vi "stimulus.vi"(7 "幅值(V)":dbl, 8 "stop frequency [Hz]":dbl, 9 "start frequency [Hz]":dbl, 10 "信号时长":dbl, 11 "Format":cluster{"Rate":i32, "Bits":i32, "Channels":u32}={"Rate"=44100, "Bits"=32, "Channels"=2}) -> (2 "Buffer size":i32, 3 "Output data":i32[][](array[numeric]))   [LabVIEW 2018]
uses:
  <vilib>/addons/_NISVFA/_Generation/SoundVib_Generation.lvlib
panel:
  in  "信号时长(s)":dbl
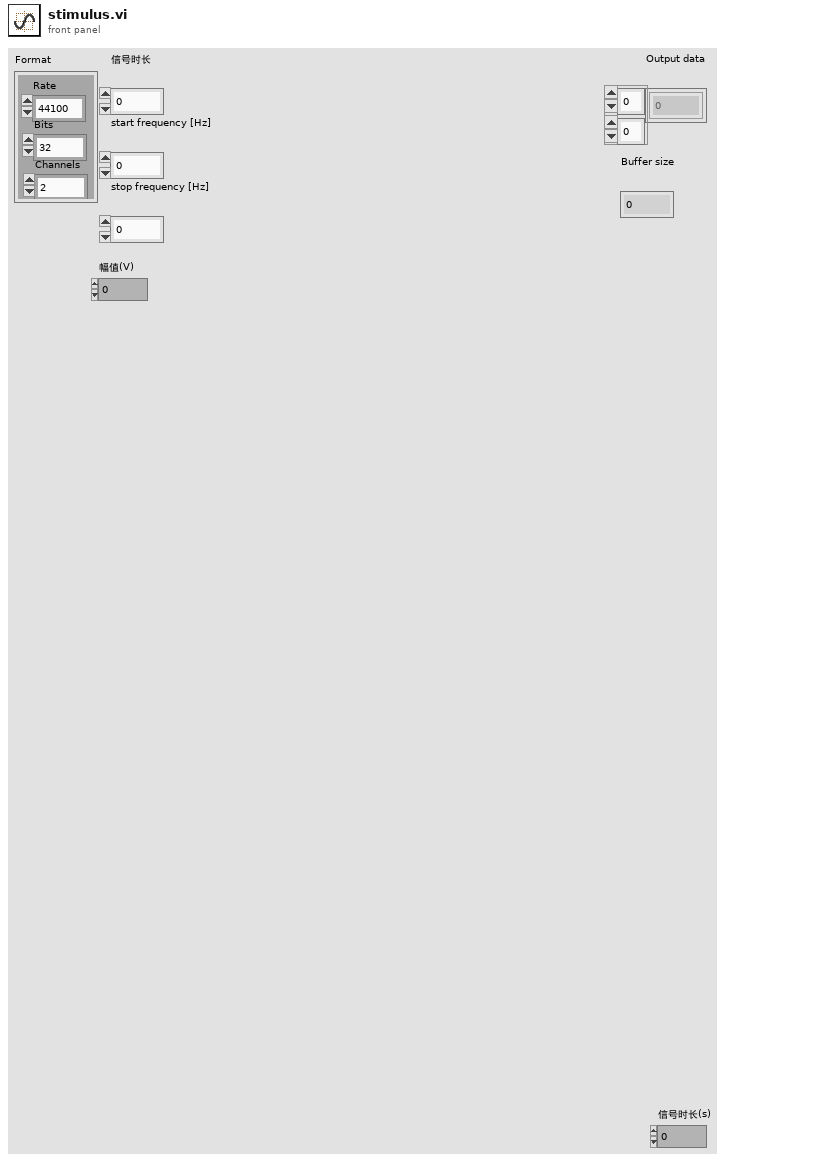
[diagram p1: front panel]
types:
  T1 = cluster{"start frequency [Hz]":dbl, "stop frequency [Hz]":dbl}
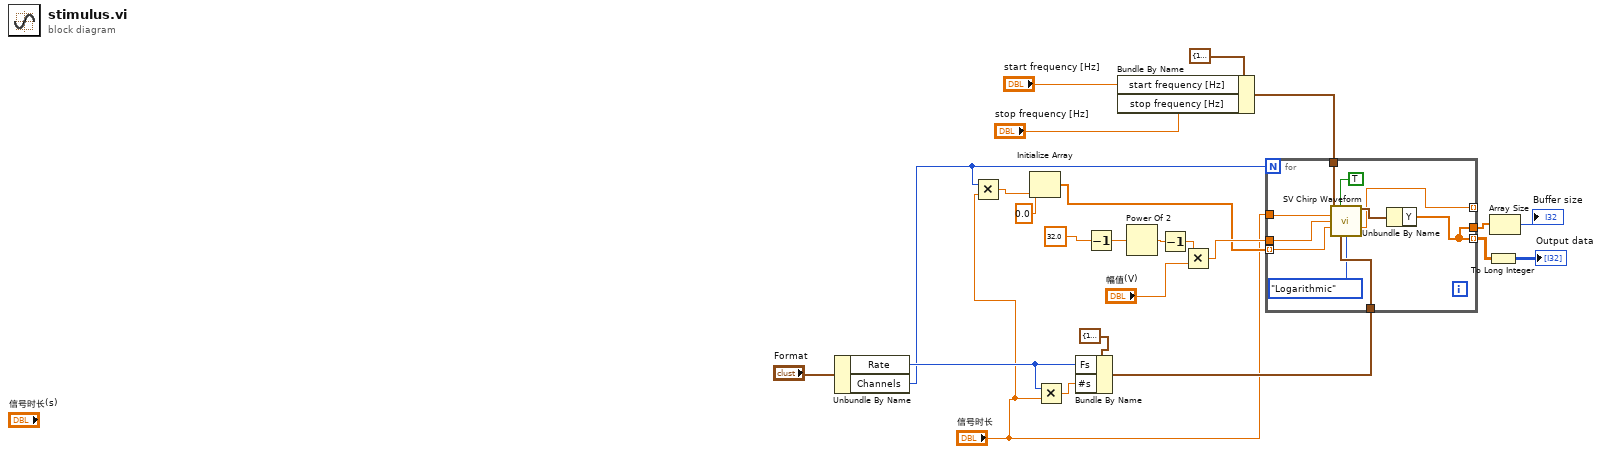
[diagram p0: block diagram]
diagram:
  n1 = Unbundle By Name("Format") -> ("Rate"=w12:i32, "Channels"=w6:u32)
  n2 = Multiply(x=w6, y="信号时长") -> (x*y=w5:dbl)
  n3 = Initialize Array(0.0 ("element"), w5) -> (w16:dbl[])
  n4 = Multiply(x=w12, y="信号时长") -> (x*y=w15:dbl)
  n5 = Bundle By Name(cluster=cluster{"Fs":dbl, "#s":dbl} {"Fs"=1000.0, "#s"=1000.0} ("sampling info"), "Fs"=w12, "#s"=w15) -> (w11:cluster{"Fs":dbl, "#s":dbl})
  n6 = Decrement(x=32.0) -> (x-1=w19:dbl)
  n7 = Bundle By Name(cluster=T1 {"start frequency [Hz]"=10.0, "stop frequency [Hz]"=10000.0} ("frequency range"), "start frequency [Hz]"="start frequency [Hz]", "stop frequency [Hz]"="stop frequency [Hz]") -> (w9:T1)
  n8 = Power Of 2(x=w19) -> (2^x=w18:dbl)
  n9 = Decrement(x=w18) -> (x-1=w24:dbl)
  n10 = Multiply(x=w24, y="幅值(V)") -> (x*y=w21:dbl)
  n11 = for {
    N: w6 -> [_]
    tunnel: [w28] -> w3 mode=indexing
    tunnel: [w33] -> _ mode=indexing
    tunnel: w16 -> [w31] mode=indexing
    tunnel: w21 -> [w30]
    tunnel: "信号时长" -> [w29]
    tunnel: [w28] -> w23
    tunnel: w11 -> [w27]
    tunnel: w9 -> [w25]
    n12 = call <vilib>:"SV Chirp Waveform.vi"("frequency range"=w25, "reset signal (F)"=TRUE ("reset signal"), "chirp duration [s]"=w29, "amplitude"=w30, "phase in [deg]"=w31, "sampling info"=w27, "frequency spacing"=enum16{"Linear", "Logarithmic"}."Logarithmic") -> ("chirp signal"=w34:waveform(dbl), "phase out [deg]"=w33:dbl)  [unwired: 6 in, 1 out]
    n13 = Unbundle By Name(w34) -> ("Y"=w28:dbl[])
  }
  n14 = To Long Integer(number=w3) -> (32bit integer=→"Output data":i32[][])
  n15 = Array Size(array=w23) -> (size(s)=→"Buffer size":i32)
